vi "Get Errno Value for Calling Thread.vi"(8 "error in (no error)":errorcluster) -> (0 "error out":errorcluster, 3 "errno":i32)   [LabVIEW 2013, in "Linux Errno.lvlib"]
doc: "This VI returns the current value of the errno variable for the calling thread. Common uses cases for this VI are in conjunction with Linux system calls, such as open(), close(), etc., which return -1 in an error state and set the value of errno for the thread rather than returning the value of errno directly."
uses:
  Linux Errno.lvlib
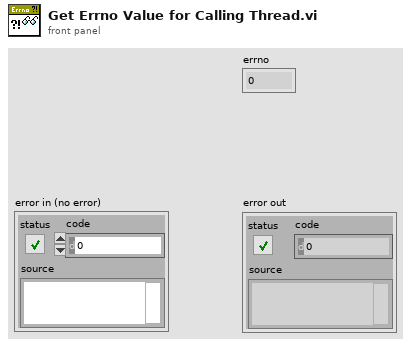
[diagram p1: front panel]
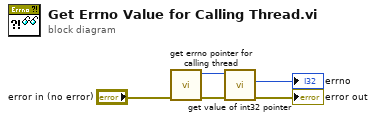
[diagram p0: block diagram]
diagram:
  n1 = call "get errno pointer for calling thread.vi"("error in (no error)"="error in (no error)") -> ("error out"=w4:errorcluster, "errno pointer"=w5:u64)  [unwired: 9 in]
  n2 = call "get value of int32 pointer.vi"("error in (no error)"=w4, "pointer in"=w5) -> ("error out"=→"error out":errorcluster, "value"=→"errno":i32)  [unwired: 7 in, 1 out]
